vi "PassFail (SubVI).vi"(0 "Type":string(combo)="Hex", 1 "Array IN":refnum<vi>, 5 "row":i32, 7 "Hex":u16 format="%.0x", 9 "ResultInput":string, 11 "error in (no error)":errorcluster, 12 "Numeric":dbl format="%#_13g") -> (6 "Test Pass(F)Fail(T)?":bool, 15 "error out":errorcluster)   [LabVIEW 2017]
uses:
  <vilib>/Utility/miscctls.llb/LVRowAndColumnTypeDef.ctl
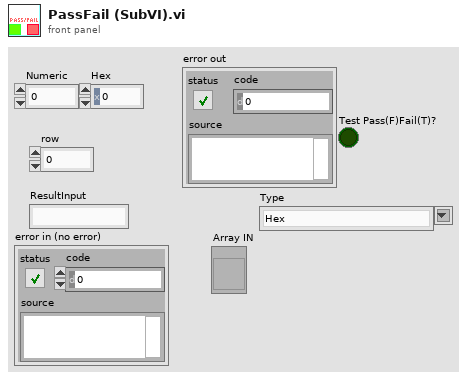
[diagram p1: front panel]
types:
  T1 = typedef "LVRowAndColumnTypeDef.ctl" = cluster{"Row":i32, "Column":i32}
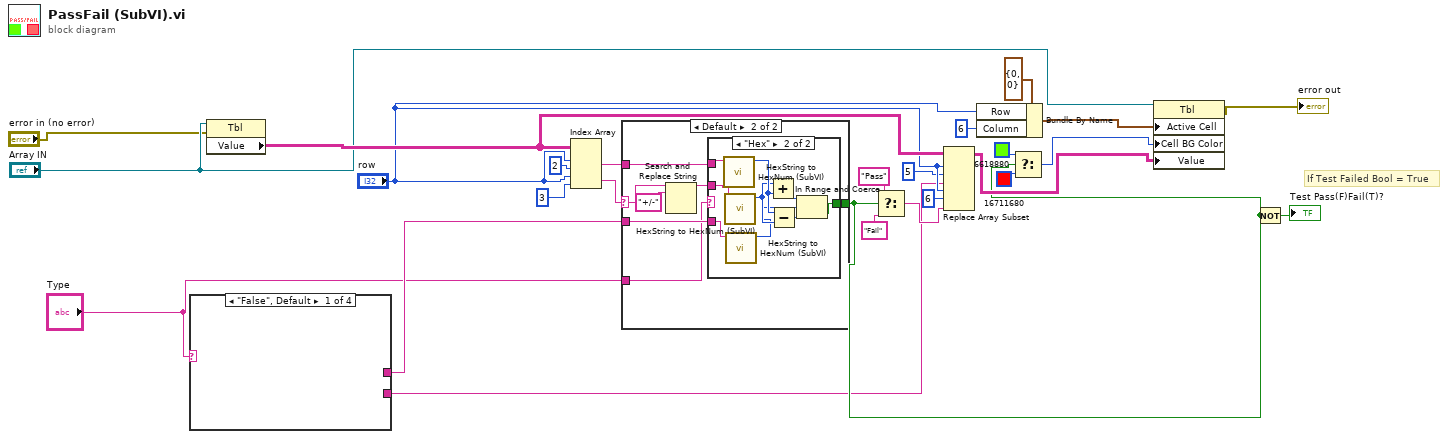
[diagram p0: block diagram]
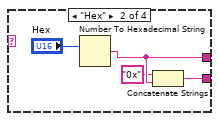
[diagram p2: hidden frame]
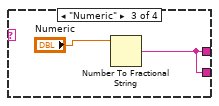
[diagram p3: hidden frame]
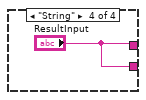
[diagram p4: hidden frame]
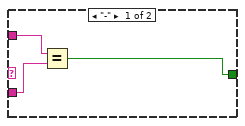
[diagram p5: hidden frame]
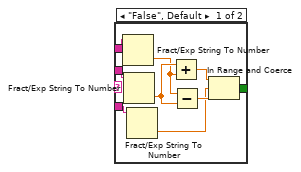
[diagram p6: hidden frame]
diagram:
  # "If Test Failed Bool = True"
  n1 = case shown="\"False\", Default" "Type" {
    tunnel: [_ w29 w31 "ResultInput"] -> w3
    tunnel: [_ w27 w31 "ResultInput"] -> w1
    frame "False", Default {
    }
    frame "Hex" {
      n2 = Number To Hexadecimal String(2:"Hex") -> (0:w29:string)  [unwired: 1 in]
      n3 = Concatenate Strings("0x" ("string"), w29) -> (w27:string)
    }
    frame "Numeric" {
      n4 = Number To Fractional String(number="Numeric") -> (F-format string=w31:string)  [unwired: 3 in]
    }
    frame "String" {
    }
  }
  n5 = property class="Tbl"(reference="Array IN", error in="error in (no error)") -> ("Value"=w16:string[][])  [unwired: 2 out]
  n6 = Index Array(array=w16, index (row) #1="row", index (col) #1=2 ("index (row)"), index (row) #2="row", index (col) #2=3 ("t")) -> (element #1=w13:string, element #2=w11:string)
  n7 = case shown="Default" w11 {
    selector: w11 -> [_ w41]
    tunnel: w3 -> [w35 w40]
    tunnel: w13 -> [w36 w39]
    tunnel: [w34 w38] -> w9
    tunnel: "Type" -> [_ w37]
    frame "-" {
      n8 = Equal?(x=w36, y=w35) -> (x = y?=w34:bool)
    }
    frame Default {
      n9 = Search and Replace String(input string=w41, search string="+/-") -> (result string=w42:string)  [unwired: 6 in, 3 out]
      n10 = case shown="\"Hex\"" w37 {
        tunnel: w42 -> [w52 w56]
        tunnel: w40 -> [w48 w54]
        tunnel: w39 -> [w46 w58]
        tunnel: [w44 w59] -> w38
        frame "False", Default {
          n11 = Fract/Exp String To Number(string=w46) -> (number=w45:dbl)  [unwired: 3 in, 1 out]
          n12 = Fract/Exp String To Number(string=w52) -> (number=w49:dbl)  [unwired: 3 in, 1 out]
          n13 = Fract/Exp String To Number(string=w48) -> (number=w47:dbl)  [unwired: 3 in, 1 out]
          n14 = Add(x=w49, y=w45) -> (x+y=w50:dbl)
          n15 = Subtract(x=w45, y=w49) -> (x-y=w51:dbl)
          n16 = In Range and Coerce(upper limit=w50, x=w47, lower limit=w51) -> (In Range?=w44:bool)  [unwired: 1 out]
        }
        frame "Hex" {
          n17 = call "HexString to HexNum (SubVI).vi"("input string"=w58) -> ("number"=w57:u32)  [unwired: 10 in]
          n18 = call "HexString to HexNum (SubVI).vi"("input string"=w56) -> ("number"=w55:u32)  [unwired: 10 in]
          n19 = call "HexString to HexNum (SubVI).vi"("input string"=w54) -> ("number"=w53:u32)  [unwired: 10 in]
          n20 = Add(x=w55, y=w57) -> (x+y=w60:u32)
          n21 = Subtract(x=w57, y=w55) -> (x-y=w61:u32)
          n22 = In Range and Coerce(upper limit=w60, x=w53, lower limit=w61) -> (In Range?=w59:bool)  [unwired: 1 out]
        }
      }
    }
  }
  n23 = Select(t="Pass", s=w9, f="Fail") -> (s? t:f=w18:string)
  n24 = Replace Array Subset(array=w16, new element #1=w1, index (row) #1="row", index (col) #1=5 ("t"), new element #2=w18, index (row) #2="row", index (col) #2=6 ("disabled index (col)")) -> (w25:string[][])
  n25 = Bundle By Name(cluster=T1 {"Row"=0, "Column"=0} ("Active Cell:Active Cell"), "Row"="row", "Column"=6) -> (w20:T1)
  n26 = Select(t=u32 6618880, s=w9, f=u32 16711680) -> (s? t:f=w24:u32)
  n27 = property class="Tbl"(reference="Array IN", "Active Cell"=w20, "Cell BG Color"=w24, "Value"=w25) -> (error out=→"error out":errorcluster)  [unwired: 1 in, 1 out]
  n28 = Not(x=w9) -> (.not. x?=→"Test Pass(F)Fail(T)?":bool)
